vi "runtime io test.vi"() -> ()   [LabVIEW 2013, in "user code tests.lvlib"]
uses:
  user code tests.lvlib
  module/execution/user tag bus module.lvclass
  module/configuration/user tag bus module configuration.lvclass/user tag bus module configuration.ctl
  <vilib>/NI/Tag Bus/tag/tag descriptor.lvclass/tag descriptor.ctl
  <vilib>/NI/Tag Bus/dictionary/data dictionary.lvclass/data dictionary.ctl
  <vilib>/NI/Tag Bus/dictionary/lookup polymorphs/locate double.vi
  <vilib>/NI/Tag Bus/table/data polymorphs/write one/write Double.vi
  <vilib>/NI/Tag Bus/tag/read tag name.vi
  module/configuration/Read state module configuration.vi
  <vilib>/NI/Tag Bus/dictionary/search/find data index.vi
  <vilib>/NI/Tag Bus/dictionary/search/search string list.vi
  <vilib>/NI/Tag Bus/dictionary/tag not found.vi
  <vilib>/NI/Tag Bus Module Framework/channel/TBM channel.lvclass
  module/configuration/user tag bus module configuration.lvclass
  <vilib>/NI/Tag Bus/dictionary/data dictionary.lvclass
  <vilib>/NI/Tag Bus/table/data table.lvlib
panel:
  out "results set":bool
  out "no error":errorcluster
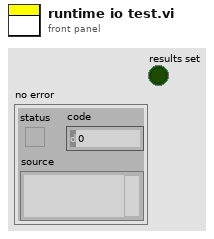
[diagram p1: front panel]
types:
  T1 = typedef "user tag bus module configuration.lvclass/state module configuration.ctl" = cluster{"fixed input":refnum<class "TBM channel.lvclass">, "fixed output":refnum<class "TBM channel.lvclass">, "initial state":u8}
  T2 = typedef "TBM channel.lvclass/data tables.ctl" = cluster{"input data":T3, "processing parameter":T3, "processing result":T3, "output data":T3}
  T3 = typedef "tag bus.lvlib/dictionary table pair.ctl" = cluster{"data dictionary":refnum<class "data dictionary.lvclass">, "data table":T4}
  T4 = typedef "tag bus.lvlib/data table.lvlib/data table.ctl" = cluster{"Double":dbl[], "Single":sgl[], "I64":i64[], "I32":i32[], "I16":i16[], "I8":i8[], "U64":u64[], "U32":u32[], "U16":u16[], "U8":u8[], "Boolean":bool[], "String":string[], "Array of Double":cluster{"DBL Array":dbl[]}[], "Array of Single":cluster{"SGL Array":sgl[]}[], "Array of I64":cluster{"I64 Array":i64[]}[], "Array of I32":cluster{"I32 Array":i32[]}[], "Array of I16":cluster{"I16 Array":i16[]}[], "Array of I8":cluster{"I8 Array":i8[]}[], "Array of U64":cluster{"U64 Array":u64[]}[], "Array of U32":cluster{"U32 Array":u32[]}[], "Array of U16":cluster{"U16 Array":u16[]}[], "Array of U8":cluster{"U8 Array":u8[]}[], "Array of Boolean":cluster{"Boolean Array":bool[]}[], "Array of String":cluster{"String Array":string[]}[]}
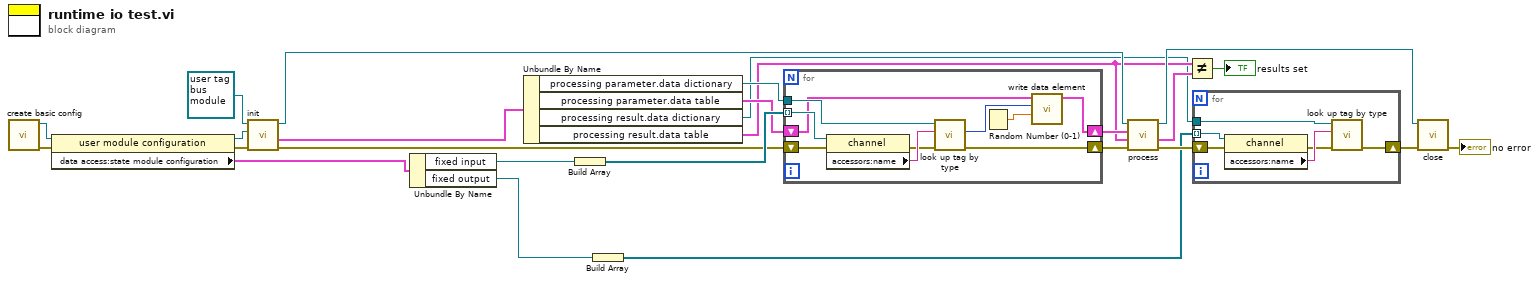
[diagram p0: block diagram]
diagram:
  n1 = call "create basic config.vi"() -> ("error out"=w22:errorcluster, "user tag bus module configuration out"=w20:refnum<class "user tag bus module configuration.lvclass">)  [unwired: 8 in, 2 out]
  n2 = property class="user module configuration"(reference=w20, error in=w22) -> (reference out=w19:refnum<class "user tag bus module configuration.lvclass">, error out=w21:errorcluster, "data access:state module configuration"=w18:T1)
  n3 = call-dynamic "init.vi"("error in"=w21, "TBM module configuration in"=w19, "tag bus configurable plugin module in"=refnum<class "user tag bus module.lvclass"> refnum ("tag bus configurable plugin module")) -> ("error out"=w11:errorcluster, "data allocations"=w24:T2, "tag bus configurable plugin module out"=w17:refnum<class "user tag bus module.lvclass">)  [unwired: 5 in, 1 out]
  n4 = Unbundle By Name(w18) -> ("fixed input"=w16:refnum<class "TBM channel.lvclass">, "fixed output"=w15:refnum<class "TBM channel.lvclass">)
  n5 = Unbundle By Name(w24) -> ("processing parameter.data dictionary"=w14:refnum<class "data dictionary.lvclass">, "processing parameter.data table"=w10:T4, "processing result.data dictionary"=w1:refnum<class "data dictionary.lvclass">, "processing result.data table"=w4:T4)
  n6 = Build Array(w16) -> (w13:refnum<class "TBM channel.lvclass">[])
  n7 = Build Array(w15) -> (w2:refnum<class "TBM channel.lvclass">[])
  n8 = for {
    tunnel: w14 -> [w35]
    tunnel: w13 -> [w34] mode=indexing
    shift-right: [w31] -> w12
    shift-left: w11 -> [w30]
    shift-right: [w28] -> w9
    shift-left: w10 -> [w29]
    n9 = property class="channel"(reference=w34, error in=w30) -> (error out=w32:errorcluster, "accessors:name"=w33:string)  [unwired: 1 out]
    n10 = call-poly <vilib>:"look up tag by type.vi"("error in"=w32, "name"=w33, "data dictionary in"=w35) -> ("error out"=w31:errorcluster, "index"=w27:i32)  [unwired: 6 in, 1 out]
    n11 = Random Number (0-1)() -> (number: 0 to 1=w26:dbl)
    n12 = call-poly <vilib>:"write data element.vi"("value"=w26, "index"=w27, "data table in"=w29) -> ("data table out"=w28:T4)  [unwired: 8 in]
  }
  n13 = call-dynamic "process.vi"("error in"=w12, "result allocation"=w4, "parameters"=w9, "module in"=w17) -> ("error out"=w7:errorcluster, "results"=w5:T4, "module out"=w8:refnum<class "user tag bus module.lvclass">)  [unwired: 4 in, 1 out]
  n14 = Not Equal?(x=w4, y=w5) -> (x != y?=→"results set":bool)
  n15 = for {
    tunnel: w2 -> [w41] mode=indexing
    shift-right: [w38] -> w6
    shift-left: w7 -> [w37]
    tunnel: w1 -> [w36]
    n16 = property class="channel"(reference=w41, error in=w37) -> (error out=w39:errorcluster, "accessors:name"=w40:string)  [unwired: 1 out]
    n17 = call-poly <vilib>:"look up tag by type.vi"("error in"=w39, "name"=w40, "data dictionary in"=w36) -> ("error out"=w38:errorcluster)  [unwired: 6 in, 2 out]
  }
  n18 = call-dynamic "close.vi"("error in"=w6, "tag bus configurable plugin module in"=w8) -> ("error out"=→"no error":errorcluster)  [unwired: 9 in]
